vi "call test.vi"() -> ()   [LabVIEW 2023]
uses:
  build/x64/Debug/MarkerLib-LabVIEW-Wrapper.dll
panel:
  in  "ZeroZone [px]":i32=-1
  in  "WinSize [px]":i32=10
  out "pointY":sgl
  out "pointX":sgl
  in  "pointY guess [px]":sgl=42.0
  in  "pointX guess [px]":sgl=52.0
  out "error out":errorcluster
  out "success":i32
  out "Intensity Graph":sgl[][](graph)
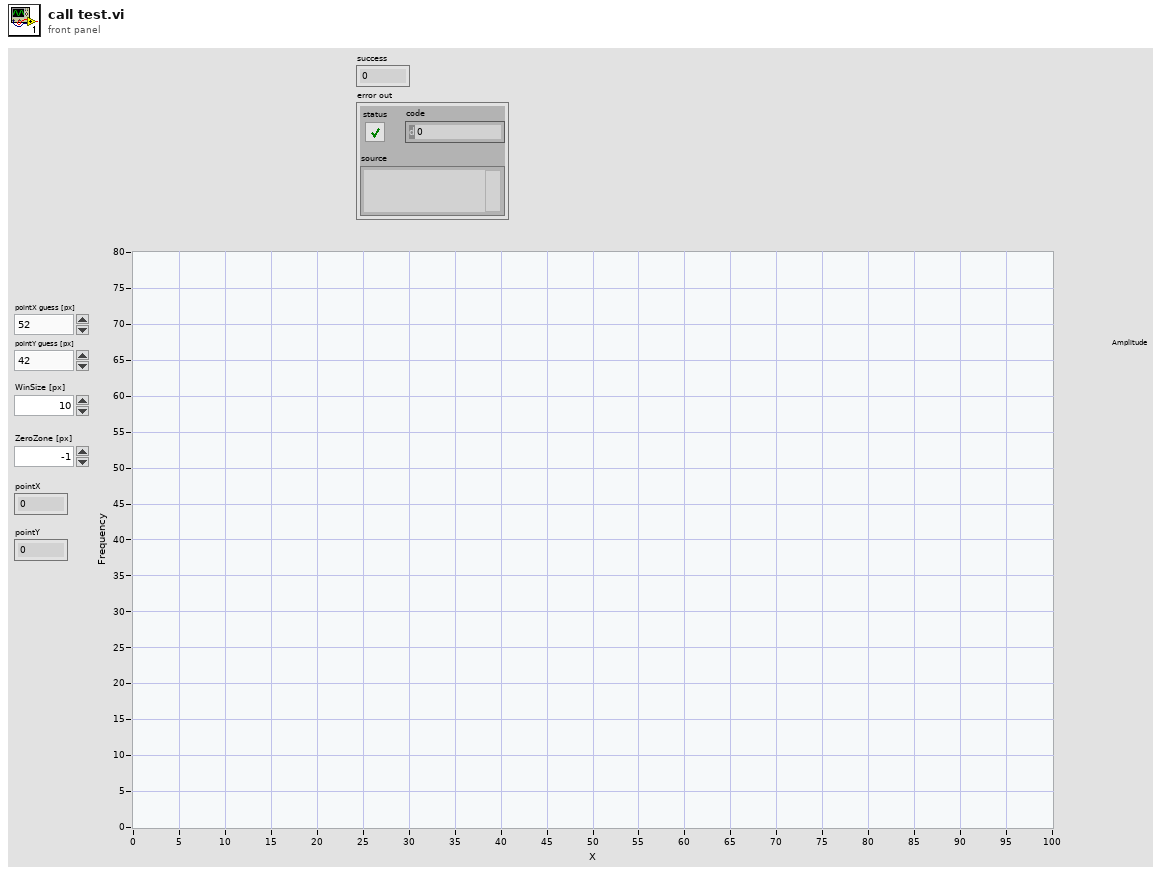
[diagram p1: front panel]
types:
  T1 = cluster{"Width":u16, "Style":enum32{"Solid", "Dash", "Dot", "DashDot", "DashDotDot"}}
  T2 = cluster{"left":i16, "top":i16, "right":i16, "bottom":i16}
  T3 = cluster{"Width":i16, "Style":enum32{"Solid", "Dash", "Dot", "DashDot", "DashDotDot"}}
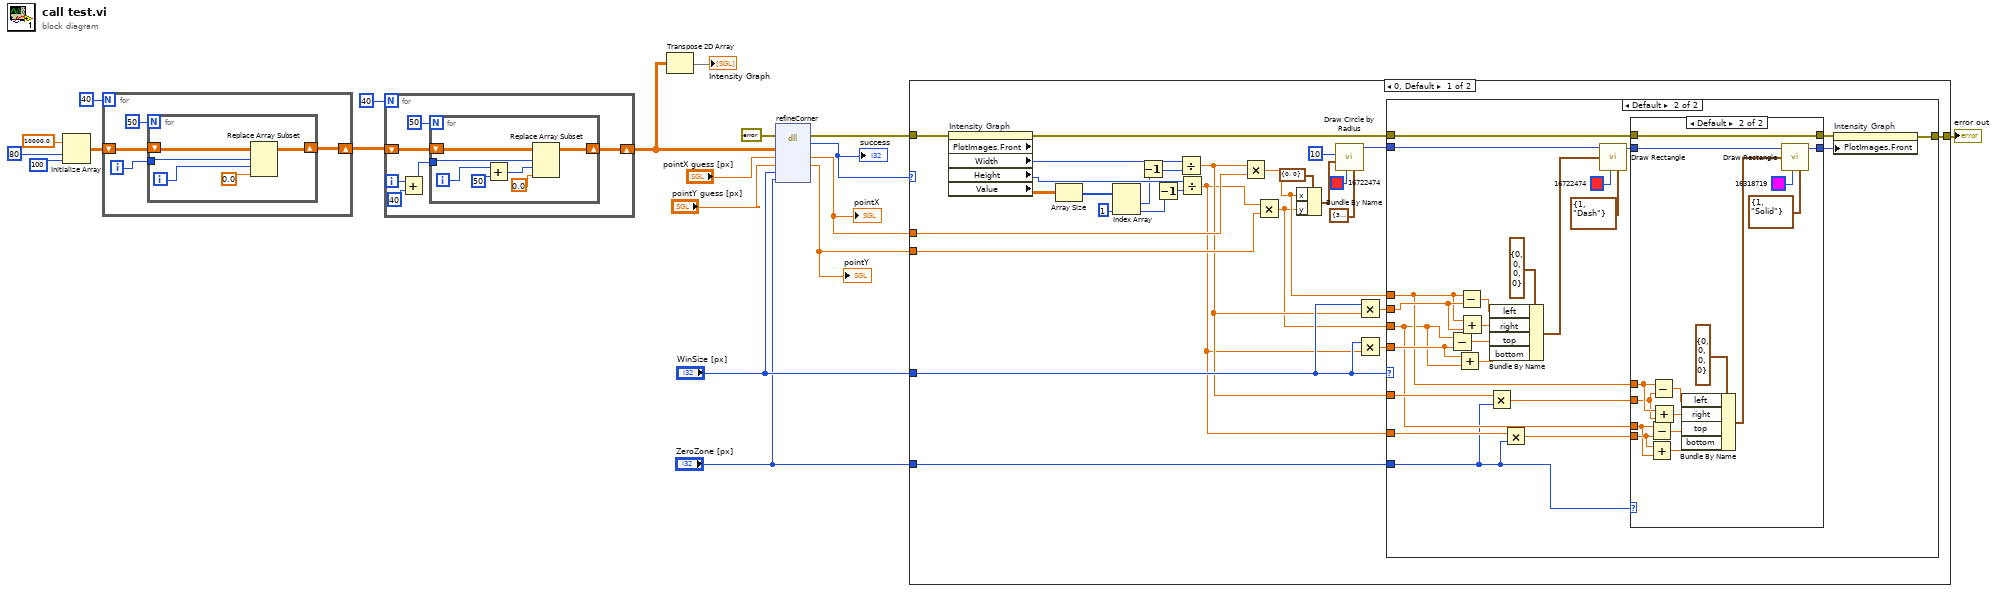
[diagram p0: block diagram]
diagram:
  n1 = Initialize Array(sgl 10000.0 ("element"), 80 ("dimension size"), 100 ("dimension size")) -> (w15:sgl[][])
  n2 = for {
    N: 40 -> [_]
    shift-right: [w23] -> w13
    shift-left: w15 -> [w21]
    i -> [w20]
    n3 = for {
      N: 50 -> [_]
      tunnel: w20 -> [w27]
      shift-right: [w25] -> w23
      shift-left: w21 -> [w28]
      i -> [w26]
      n4 = Replace Array Subset(array=w28, new element=sgl 0.0 ("new element/subarray"), index (row)=w27, index (col)=w26) -> (w25:sgl[][])
    }
  }
  n5 = for {
    N: 40 -> [_]
    shift-right: [w34] -> w11
    shift-left: w13 -> [w32]
    i -> [w31]
    n6 = Add(x=w31, y=40) -> (x+y=w29:i32)
    n7 = for {
      N: 50 -> [_]
      tunnel: w29 -> [w40]
      shift-right: [w38] -> w34
      shift-left: w32 -> [w41]
      i -> [w39]
      n8 = Add(x=w39, y=50) -> (x+y=w37:i32)
      n9 = Replace Array Subset(array=w41, new element=sgl 0.0 ("new element/subarray"), index (row)=w40, index (col)=w37) -> (w38:sgl[][])
    }
  }
  n10 = Transpose 2D Array(2D array=w11) -> (transposed array=→"Intensity Graph":sgl[][])
  n11 = dll-call lib="D:/git/MarkerLib-LabVIEW-Wrapper/build/x64/Debug/MarkerLib-LabVIEW-Wrapper.dll" fn="refineCorner"(error in=errorcluster {"status"=FALSE, "code"=0, "source"=""} ("error in (no error)"), "image"=w11, "pointX"="pointX guess [px]", "pointY"="pointY guess [px]", "winSize"="WinSize [px]", "zeroZone"="ZeroZone [px]") -> (error out=w9:errorcluster, "success"=w3:i32, "pointX"=w6:sgl, "pointY"=w7:sgl)  [unwired: 5 in, 1 out]
  "success" <- w3
  "pointY" <- w7
  "pointX" <- w6
  n12 = case shown="0, Default" w3 {
    tunnel: w9 -> [w69 w111]
    tunnel: [w63 w111] -> w8
    tunnel: w7 -> [w59 _]
    tunnel: w6 -> [w58 _]
    tunnel: "WinSize [px]" -> [w47 _]
    tunnel: "ZeroZone [px]" -> [w42 _]
    frame 0, Default {
      n13 = property on="Intensity Graph" class="IntGraph (strict)" props=["PlotImages.Front", "Width", "Height", "Value"](error in=w69) -> (error out=w64:errorcluster, "Width"=w61:u32, "Height"=w60:u32, "Value"=w56:sgl[][])  [unwired: 1 in, 2 out]
      n14 = Array Size(array=w56) -> (size(s)=w55:i32[])
      n15 = Index Array(array=w55, index #2=1 ("index")) -> (element #1=w54:i32, element #2=w53:i32)  [unwired: 1 in]
      n16 = Decrement(x=w54) -> (x-1=w50:i32)
      n17 = Decrement(x=w53) -> (x-1=w51:i32)
      n18 = Divide(x=w61, y=w50) -> (x/y=w46:dbl)
      n19 = Divide(x=w60, y=w51) -> (x/y=w45:dbl)
      n20 = Multiply(x=w46, y=w58) -> (x*y=w44:dbl)
      n21 = Multiply(x=w45, y=w59) -> (x*y=w43:dbl)
      n22 = Bundle By Name(cluster=cluster{"x":i16, "y":i16} {"x"=0, "y"=0} ("point(x,y)"), "x"=w44, "y"=w43) -> (w67:cluster{"x":i16, "y":i16})
      n23 = call <vilib>:"Draw Circle by Radius.vi"("pen"=T1 {"Width"=3, "Style"=enum."Dot"}, "color(black)"=u32 16722474, "pixel center"=w67, "radius"=i16 10) -> ("new picture"=w57:picture)  [unwired: 7 in]
      n24 = Multiply(x=w47, y=w46) -> (x*y=w49:dbl)
      n25 = Multiply(x=w47, y=w45) -> (x*y=w48:dbl)
      n26 = case shown="Default" w47 {
        tunnel: w64 -> [w70 w79]
        tunnel: [w70 w93] -> w63
        tunnel: w57 -> [_ w92]
        tunnel: w44 -> [_ w75]
        tunnel: w49 -> [_ w82]
        tunnel: w43 -> [_ w72]
        tunnel: w48 -> [_ w83]
        tunnel: w46 -> [_ w77]
        tunnel: w45 -> [_ w76]
        tunnel: w42 -> [_ w71]
        frame -1 {
        }
        frame Default {
          n27 = Subtract(x=w72, y=w83) -> (x-y=w85:dbl)
          n28 = Add(x=w83, y=w72) -> (x+y=w84:dbl)
          n29 = Subtract(x=w75, y=w82) -> (x-y=w87:dbl)
          n30 = Add(x=w75, y=w82) -> (x+y=w86:dbl)
          n31 = Multiply(x=w77, y=w71) -> (x*y=w74:dbl)
          n32 = Bundle By Name(cluster=T2 {"left"=0, "top"=0, "right"=0, "bottom"=0} ("rect"), "left"=w87, "right"=w86, "top"=w85, "bottom"=w84) -> (w88:T2)
          n33 = Multiply(x=w76, y=w71) -> (x*y=w73:dbl)
          n34 = call <vilib>:"Draw Rectangle.vi"("picture"=w92, "rect"=w88, "color(black)"=u32 16722474, "pen"=T1 {"Width"=1, "Style"=enum."Dash"}) -> ("new picture"=w81:picture)  [unwired: 5 in]
          n35 = case shown="Default" w71 {
            tunnel: w81 -> [w94 w110]
            tunnel: [w94 w109] -> w80
            tunnel: w79 -> [w95 w108]
            tunnel: [w95 w108] -> w78
            tunnel: w75 -> [_ w99]
            tunnel: w74 -> [_ w98]
            tunnel: w73 -> [_ w97]
            tunnel: w72 -> [_ w96]
            frame -1 {
            }
            frame Default {
              n36 = Subtract(x=w96, y=w97) -> (x-y=w103:dbl)
              n37 = Add(x=w97, y=w96) -> (x+y=w102:dbl)
              n38 = Subtract(x=w99, y=w98) -> (x-y=w105:dbl)
              n39 = Add(x=w99, y=w98) -> (x+y=w104:dbl)
              n40 = Bundle By Name(cluster=T2 {"left"=0, "top"=0, "right"=0, "bottom"=0} ("rect"), "left"=w105, "right"=w104, "top"=w103, "bottom"=w102) -> (w101:T2)
              n41 = call <vilib>:"Draw Rectangle.vi"("picture"=w110, "rect"=w101, "color(black)"=u32 16318719, "pen"=T3 {"Width"=1, "Style"=enum."Solid"}) -> ("new picture"=w109:picture)  [unwired: 5 in]
            }
          }
          n42 = property on="Intensity Graph" class="IntGraph (strict)"(error in=w78, "PlotImages.Front"=w80) -> (error out=w93:errorcluster)  [unwired: 1 in, 1 out]
        }
      }
    }
    frame 1 {
    }
  }
  "error out" <- w8
